vi "Filepath 2 Hidden Files.vi"(0 "DataFilePath":path, 2 "Enum":enum16{"Data", "Stats", "Specs"}(ring)) -> (4 "HiddenFilePath":path)   [LabVIEW 2013]
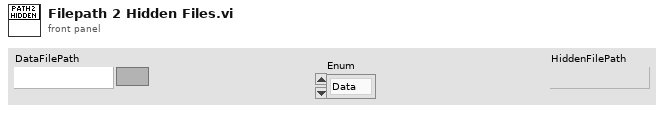
[diagram p1: front panel]
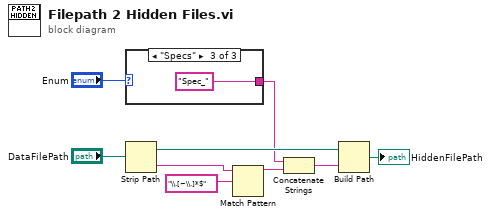
[diagram p0: block diagram]
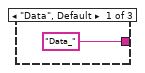
[diagram p2: hidden frame]
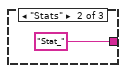
[diagram p3: hidden frame]
diagram:
  n1 = case shown="\"Specs\"" "Enum" {
    tunnel: ["Data_" ("string") "Stat_" ("string") "Spec_" ("string")] -> w2
    frame "Data", Default {
    }
    frame "Stats" {
    }
    frame "Specs" {
    }
  }
  n2 = Strip Path(path="DataFilePath") -> (stripped path=w6:path, name=w8:string)
  n3 = Match Pattern(string=w8, regular expression="\\.[~\\.]*$") -> (before substring=w1:string)  [unwired: 4 out]
  n4 = Concatenate Strings(w2, w1) -> (w5:string)
  n5 = Build Path(base path=w6, name or relative path=w5) -> (appended path=→"HiddenFilePath":path)
